vi "fpga_Fixed Array.vi"(1 "Array":T1(array[cluster])=[{"frequency"=0.0, "timestamp"=0.0}, {"frequency"=0.0, "timestamp"=0.0}, {"frequency"=0.0, "timestamp"=0.0}, {"frequency"=0.0, "timestamp"=0.0}, {"frequency"=0.0, "timestamp"=0.0}, {"frequency"=0.0, "timestamp"=0.0}, {"frequency"=0.0, "timestamp"=0.0}]) -> (0 "Array 2":T1(array[cluster]))   [LabVIEW 2011, in "NI_EP_PMU_FPGA.lvlib"]
uses:
  <vilib>/addons/Electrical Power/PMU/NI_EP_PMU_FPGA.lvlib
types:
  T1 = cluster{"frequency":fxp<+,32,8>, "timestamp":fxp<+,64,32>}[]
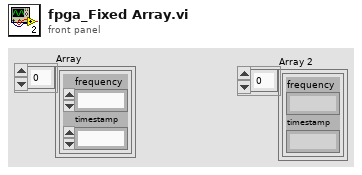
[diagram p1: front panel]
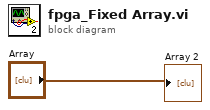
[diagram p0: block diagram]
diagram:
  "Array 2" <- "Array"
